vi "LvMPDC_SUB_SetPlaybackOption.vi"(6 "timeout_ms":i32=25000, 8 "error in (no error)":errorcluster, 9 "ReadBytes":i32=1024, 10 "volume":T1, 11 "Connect ID":refnum<k5>) -> (0 "error out":errorcluster, 3 "Connect ID out":refnum<k5>)   [LabVIEW 2012]
uses:
  LvMPDC_Typdef_PlaybackOption.ctl
panel:
  # "LvMPDC:: CMD SetPlaybackOption"
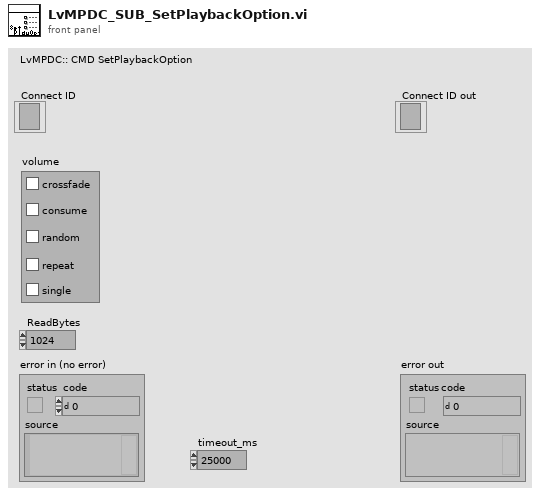
[diagram p1: front panel]
types:
  T1 = typedef "LvMPDC_Typdef_PlaybackOption.ctl" = cluster{"chk crossfade":bool, "chk consume":bool, "chk random":bool, "chk repeat":bool, "chk single":bool}
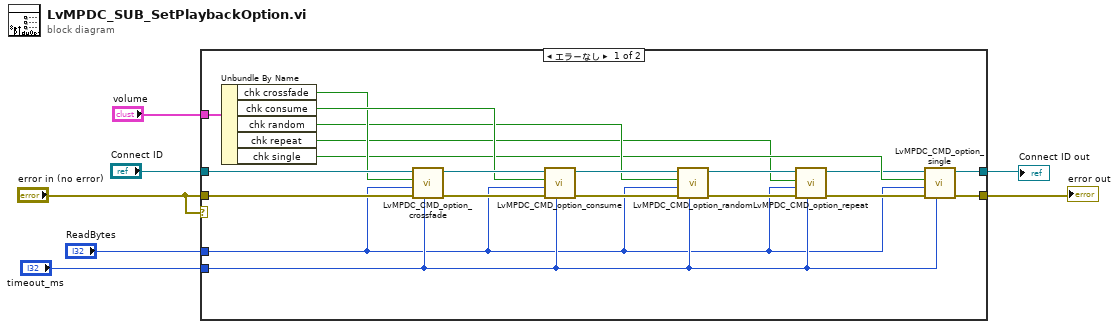
[diagram p0: block diagram]
diagram:
  n1 = case shown="エラーなし" "error in (no error)" {
    tunnel: "Connect ID" -> [w25 w28]
    tunnel: "error in (no error)" -> [w19 w27]
    tunnel: [w20 w28] -> w6
    tunnel: [w15 w27] -> w5
    tunnel: "timeout_ms" -> [w9 _]
    tunnel: "ReadBytes" -> [w8 _]
    tunnel: "volume" -> [w26 _]
    frame No Error {
      n2 = Unbundle By Name(w26) -> ("chk crossfade"=w14:bool, "chk consume"=w23:bool, "chk random"=w13:bool, "chk repeat"=w10:bool, "chk single"=w12:bool)
      n3 = call "LvMPDC_CMD_option_crossfade.vi"("timeout_ms"=w9, "error in (no error)"=w19, "ReadBytes"=w8, "sw"=w14, "Connect ID"=w25) -> ("error out"=w18:errorcluster, "Connect ID out"=w24:refnum<k5>)  [unwired: 5 in]
      n4 = call "LvMPDC_CMD_option_consume.vi"("timeout_ms"=w9, "error in (no error)"=w18, "ReadBytes"=w8, "sw"=w23, "Connect ID"=w24) -> ("error out"=w17:errorcluster, "Connect ID out"=w22:refnum<k5>)  [unwired: 5 in]
      n5 = call "LvMPDC_CMD_option_random.vi"("timeout_ms"=w9, "error in (no error)"=w17, "ReadBytes"=w8, "sw"=w13, "Connect ID"=w22) -> ("error out"=w16:errorcluster, "Connect ID out"=w21:refnum<k5>)  [unwired: 5 in]
      n6 = call "LvMPDC_CMD_option_repeat.vi"("timeout_ms"=w9, "ReadBytes"=w8, "sw"=w10, "Connect ID"=w21) -> ("Connect ID out"=w11:refnum<k5>)  [unwired: 6 in, 1 out]
      n7 = call "LvMPDC_CMD_option_single.vi"("timeout_ms"=w9, "error in (no error)"=w16, "ReadBytes"=w8, "sw"=w12, "Connect ID"=w11) -> ("error out"=w15:errorcluster, "Connect ID out"=w20:refnum<k5>)  [unwired: 5 in]
    }
    frame Error {
    }
  }
  "Connect ID out" <- w6
  "error out" <- w5
